vi "URAPICompile.vi"(1 "Comments?":bool, 2 "Script":string) -> (0 "trimmed script":string)   [LabVIEW 2012]
panel:
  out "Array":string[](array[string])
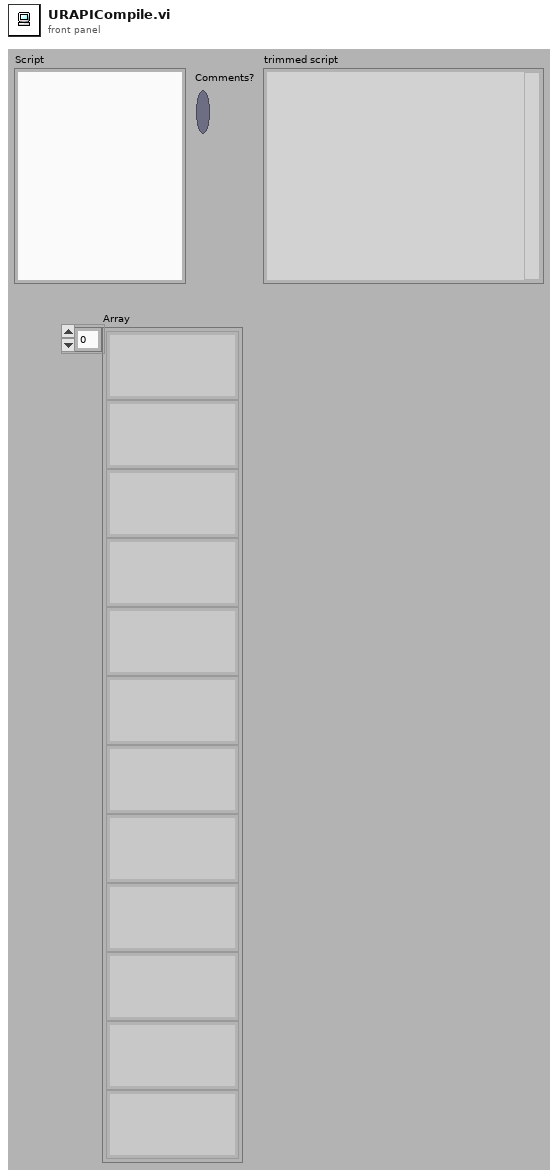
[diagram p1: front panel]
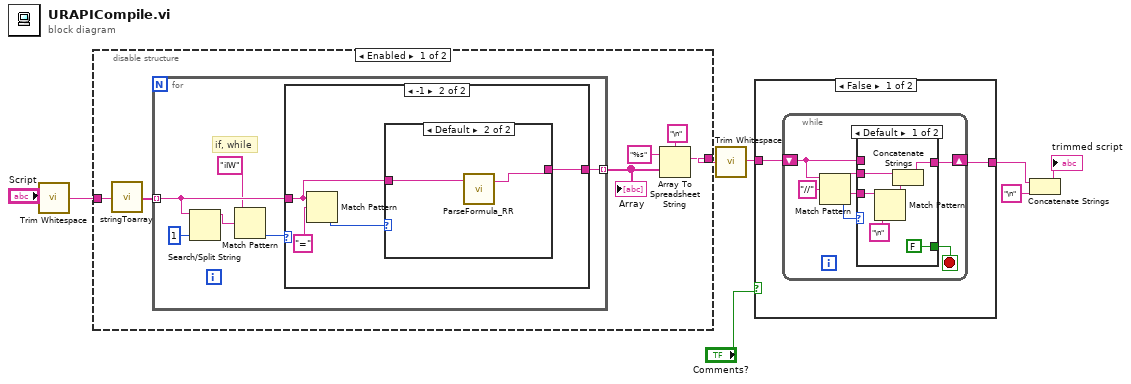
[diagram p0: block diagram]
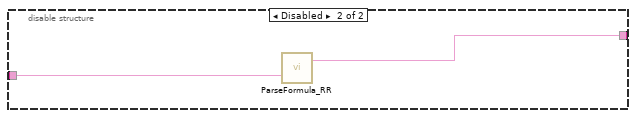
[diagram p4: hidden frame]
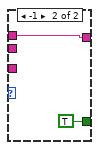
[diagram p5: hidden frame]
diagram:
  n1 = call <vilib>:"Trim Whitespace.vi"("string"="Script") -> ("trimmed string"=w1:string)  [unwired: 1 in]
  n2 = disable-structure shown="Enabled" {
    disable-tunnel: w1 -> [w10 w30]
    disable-tunnel: [w9 w29] -> w2
    frame Enabled {
      n3 = call <userlib>:"stringToarray.vi"("String"=w10) -> ("Array"=w13:string[])
      n4 = for {
        tunnel: w13 -> [w19] mode=indexing
        tunnel: [w20] -> w14 mode=indexing
        # "if, while"
        n5 = Search/Split String(string=w19, offset (0)=1) -> (substring before match=w17:string)  [unwired: 1 in, 2 out]
        n6 = Match Pattern(string="iIW" ("search string/char (-)"), regular expression=w17) -> (offset past match=w15:i32)  [unwired: 1 in, 3 out]
        n7 = case shown="-1" w15 {
          tunnel: [w21 w23] -> w20
          tunnel: w19 -> [w21 w22]
          frame 0, Default {
          }
          frame -1 {
            n8 = Match Pattern(string=w22, regular expression="=") -> (offset past match=w24:i32)  [unwired: 1 in, 3 out]
            n9 = case shown="Default" w24 {
              tunnel: [w26 w27] -> w23
              tunnel: w22 -> [w26 w28]
              frame -1 {
              }
              frame Default {
                n10 = call <userlib>:"ParseFormula_RR.vi"("Script"=w28) -> ("URAPI"=w27:string)  [unwired: 2 in]
              }
            }
          }
        }
      }
      "Array" <- w14
      n11 = Array To Spreadsheet String(delimiter (Tab)="\n", array=w14, 3:"%s" ("format string")) -> (spreadsheet string=w9:string)
    }
    frame Disabled {
      n12 = call <userlib>:"ParseFormula_RR.vi"("Script"=w30) -> ("URAPI"=w29:string)  [unwired: 2 in]
    }
  }
  n13 = call <vilib>:"Trim Whitespace.vi"("string"=w2) -> ("trimmed string"=w7:string)  [unwired: 1 in]
  n14 = case shown="False" "Comments?" {
    tunnel: w7 -> [w32 w48]
    tunnel: [w31 w48] -> w5
    frame False {
      n15 = while {
        shift-right: [w39] -> w31
        shift-left: w32 -> [w36]
        stop <- w35 stop-if-true
        n16 = Match Pattern(string=w36, regular expression="//") -> (before substring=w33:string, after substring=w34:string, offset past match=w37:i32)  [unwired: 1 in, 1 out]
        n17 = case shown="Default" w37 {
          tunnel: [w43 w46] -> w39
          tunnel: w36 -> [_ w46]
          tunnel: [FALSE TRUE] -> w35
          tunnel: w34 -> [w45 _]
          tunnel: w33 -> [w42 _]
          frame Default {
            n18 = Match Pattern(string=w45, regular expression="\n" ("delimiter (Tab)")) -> (after substring=w41:string)  [unwired: 1 in, 3 out]
            n19 = Concatenate Strings(w42, w41) -> (w43:string)
          }
          frame -1 {
          }
        }
      }
    }
    frame True {
    }
  }
  n20 = Concatenate Strings(w5, "\n" ("command")) -> (→"trimmed script":string)
